vi "Gear Intake Auto Loop.vi"(0 "Gear Load Height":dbl, 1 "Idle Height":dbl, 5 "Intake Speed":dbl, 7 "Intake Gear?":bool, 9 "Outake Speed":dbl, 11 "Set Time":dbl, 12 "Ball?":bool) -> (4 "Gear States":T1, 6 "Intake Height":dbl, 10 "Roller Speed":dbl)   [LabVIEW 2016]
uses:
  Common Code/Gear States.ctl
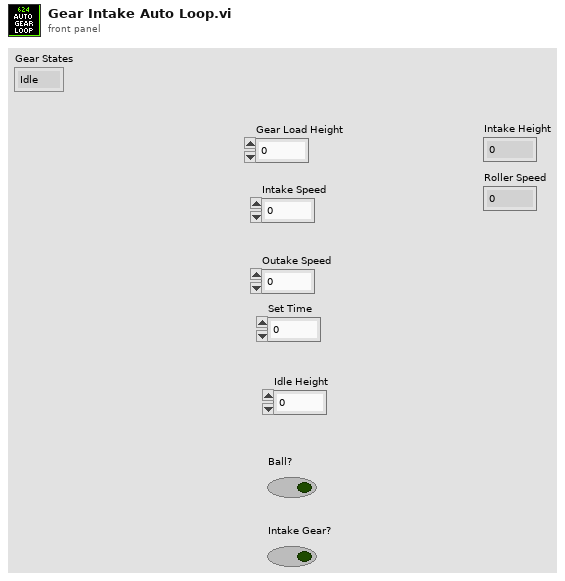
[diagram p1: front panel]
types:
  T1 = typedef "Gear States.ctl" = enum16{"Idle", "Warmup", "Load", "Set"}
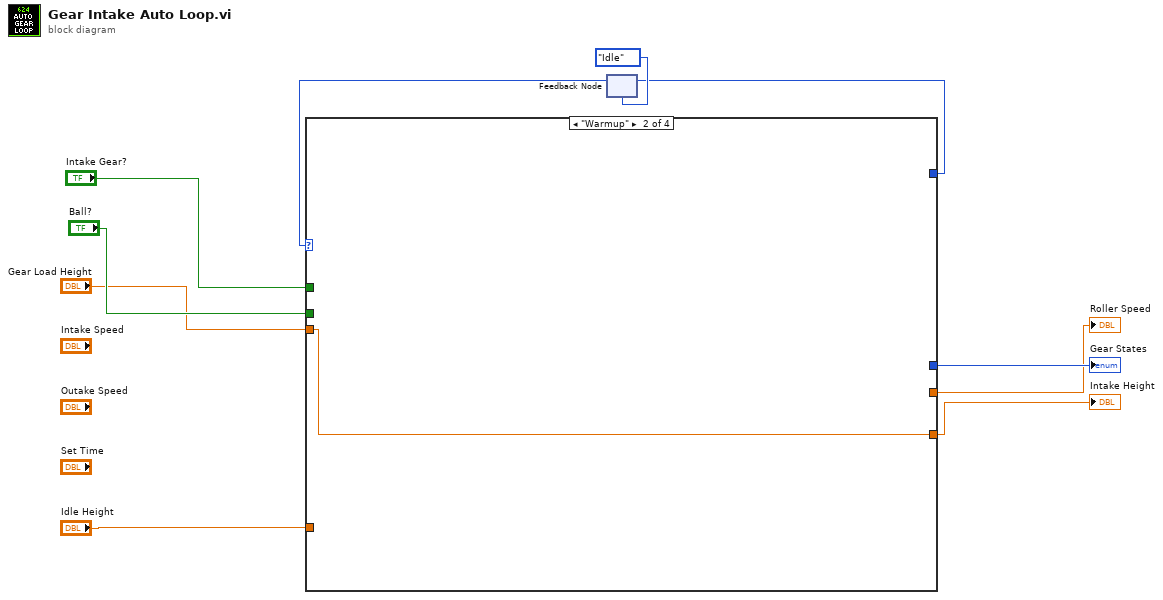
[diagram p0: block diagram]
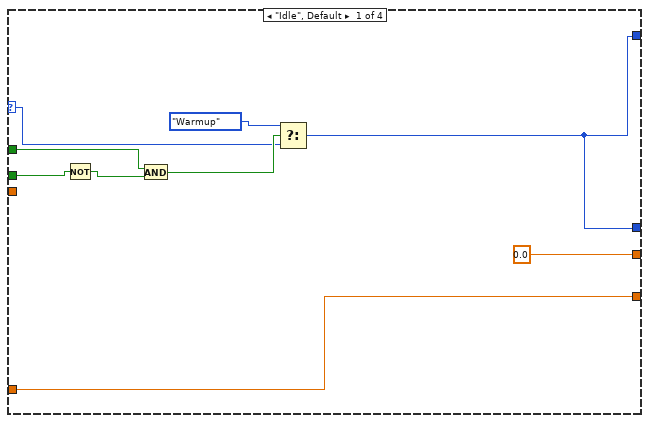
[diagram p2: hidden frame]
diagram:
  n1 = feedback #1(Gear_States."Idle" ("Gear States")) -> (w8:T1)
  n2 = case shown="\"Warmup\"" w8 {
    selector: w8 -> [w14 _ _ _]
    tunnel: [w13 _ _ _] -> w9
    tunnel: "Ball?" -> [w17 _ _ _]
    tunnel: "Intake Gear?" -> [w19 _ _ _]
    tunnel: [w13 _ _ _] -> w5
    tunnel: [w12 w20 _ _] -> w3
    tunnel: "Idle Height" -> [w12 _ _ _]
    tunnel: [0.0 _ _ _] -> w2
    tunnel: "Gear Load Height" -> [_ w20 _ _]
    frame "Idle", Default {
      n3 = Not(x=w17) -> (.not. x?=w16:bool)
      n4 = And(x=w19, y=w16) -> (x .and. y?=w18:bool)
      n5 = Select(t=Gear_States."Warmup" ("Gear States"), s=w18, f=w14) -> (s? t:f=w13:T1)
    }
    frame "Warmup" {
    }
    frame "Load" {
    }
    frame "Set" {
    }
  }
  "Gear States" <- w5
  "Intake Height" <- w3
  "Roller Speed" <- w2
  n6 = feedback-in #1(w9) -> ()
